vi "Pre Launch Init.vi"(11 "Capillary Line in":refnum<class "Capillary Line.lvclass">) -> (0 "error out":errorcluster, 3 "Capillary Line out":refnum<class "Capillary Line.lvclass">)   [LabVIEW 2015, in "cRIO-Carbondioxide.lvlib" / "CO2-Actor.lvlib" / "Capillary Line.lvclass"]
doc: "(<B>Filename</B>: Actor Framework.lvlib:Actor.lvclass:Pre Launch Init.vi)\n\nDefines behavior that occurs after the Launch Actor method is invoked but before the actor's Actor Core method begins running.\n\nThe Pre Launch Init method is guaranteed to finish before the Launch Actor method returns to its caller and before the actor itself receives any messages. Any references that the Pre Launch Init method obtains are guaranteed to have the same lifetime as the actor itself. Any errors that the Pre Launch Init method returns will abort the launch.\n\nBy default, this method does nothing. A descendant class may override it to define behavior."
uses:
  Capillary Line.lvclass
  Capillary Line.lvclass/Capillary Line.ctl
  <vilib>/ActorFramework/Actor/Actor.lvclass/Actor.ctl
  <vilib>/ActorFramework/Message Enqueuer/Message Enqueuer.lvclass/Message Enqueuer.ctl
  <vilib>/ActorFramework/Actor/Read Self Enqueuer.vi
  <vilib>/ActorFramework/Message Enqueuer/Enqueue.vi
  <vilib>/ActorFramework/Message Enqueuer/Init from Existing Queue.vi
  <vilib>/ActorFramework/Message Priority Queue/Priority Enqueue.vi
  CO2 Actor/CO2 Actor.lvclass
  CO2 Actor Messages/Launch Nested Actors Msg/Launch Nested Actors Msg.lvclass
  <vilib>/ActorFramework/Message Enqueuer/Message Enqueuer.lvclass
  <vilib>/ActorFramework/Actor/Actor.lvclass
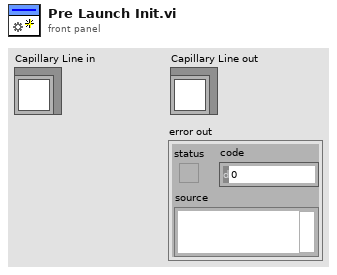
[diagram p1: front panel]
types:
  T1 = typedef "Sample Container.ctl" = cluster{"Sample In":refnum<k21>, "Sample Name":refnum<k21>, "Ti Cathode":refnum<k21>, "SampleQ":refnum<queue>}
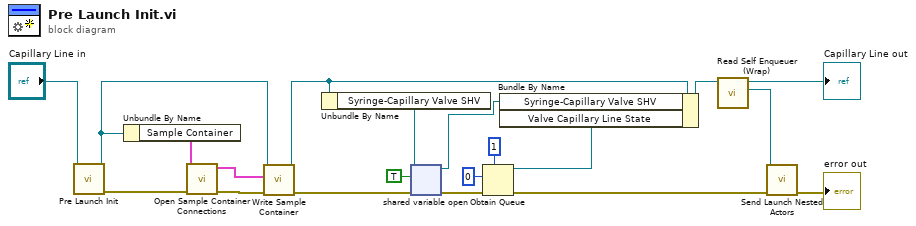
[diagram p0: block diagram]
diagram:
  n1 = call-parent "Pre Launch Init.vi"("CO2 Actor in"="Capillary Line in") -> ("error out"=w9:errorcluster, "CO2 Actor out"=w7:refnum<class "Capillary Line.lvclass">)  [unwired: 9 in]
  n2 = Unbundle By Name(w7) -> ("Sample Container"=w8:T1)
  n3 = call "Open Sample Container Connections.vi"("error in (no error)"=w9, "Container in"=w8) -> ("error out"=w19:errorcluster, "Container out"=w10:T1)  [unwired: 8 in]
  n4 = call "Write Sample Container.vi"("error in (no error)"=w19, "Sample Container"=w10, "Capillary Line in"=w7) -> ("error out"=w17:errorcluster, "Capillary Line out"=w18:refnum<class "Capillary Line.lvclass">)  [unwired: 7 in]
  n5 = Unbundle By Name(w18) -> ("Syringe-Capillary Valve SHV"=w16:refnum<k21>)
  n6 = shared-variable-open(w16, w17, TRUE) -> (w5:refnum<k21>, w3:errorcluster)  [unwired: 1 in]
  n7 = Obtain Queue(max queue size (-1, unlimited)=1, element data type=u16 0 ("Valve Capillary Valve State"), error in (no error)=w3) -> (queue out=w1:refnum<queue>, error out=w2:errorcluster)  [unwired: 2 in, 1 out]
  n8 = Bundle By Name(cluster=w18, "Syringe-Capillary Valve SHV"=w5, "Valve Capillary Line State"=w1) -> (w14:refnum<class "Capillary Line.lvclass">)
  n9 = call "Read Self Enqueuer (Wrap).vi"("CO2 Actor in"=w14) -> ("Actor Framework:Message Enqueuer"=w11:refnum<class "Message Enqueuer.lvclass">, "CO2 Actor out"=→"Capillary Line out":refnum<class "Capillary Line.lvclass">)  [unwired: 9 in]
  n10 = call "Send Launch Nested Actors.vi"("error in (no error)"=w2, "Message Enqueuer"=w11) -> ("error out"=→"error out":errorcluster)  [unwired: 8 in, 1 out]
